vi "Textures Control.vi"(10 "Trial In Progress IN":T1, 11 "Trial Fraction IN":dbl) -> (2 "Left Texture Control":bool, 3 "Right Texture Control":bool)   [LabVIEW 2018]
uses:
  controls/Trial Config Settings.ctl
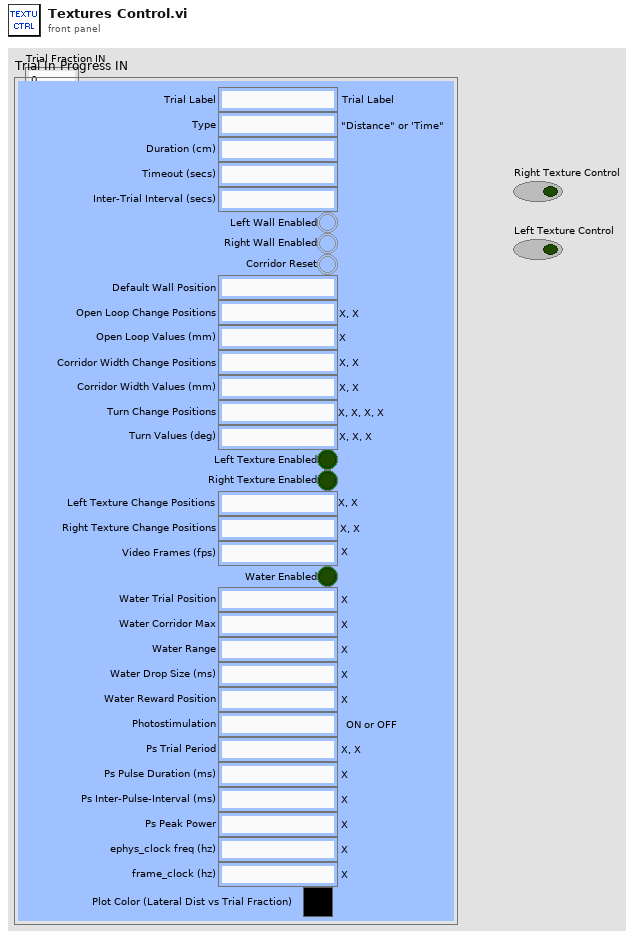
[diagram p1: front panel]
types:
  T1 = typedef "Trial Config Settings.ctl" = cluster{"Trial Label":string, "Type":string, "Timeout (secs)":string, "Inter-Trial Interval (secs)":string, "Left Wall Enabled":bool, "Right Wall Enabled":bool, "Corridor Reset":bool, "Default Wall Position":string, "Open Loop Change Positions":string, "Open Loop Values (mm)":string, "Corridor Width Change Positions":string, "Corridor Width Values (mm) ":string, "Turn Change Positions":string, "Turn Values (deg)":string, "Left Texture Change Positions":string, "Right Texture Change Positions":string, "Video Frames (fps)":string, "Water Enabled":bool, "Water Trial Position":string, "Photostimulation":string, "Water Corridor Max":string, "Water Range":string, "Water Drop Size (ms)":string, "Water Reward Position":string, "Duration (cm)":string, "Left Texture Enabled":bool, "Right Texture Enabled":bool, "Ps Trial Period":string, "Ps Inter-Pulse-Interval (ms)":string, "Ps Peak Power":string, "Ps Pulse Duration (ms)":string, "ephys_clock freq (hz)":string, "frame_clock (hz)":string, "Plot Color (Lateral Dist vs Trial Fraction)":u32}
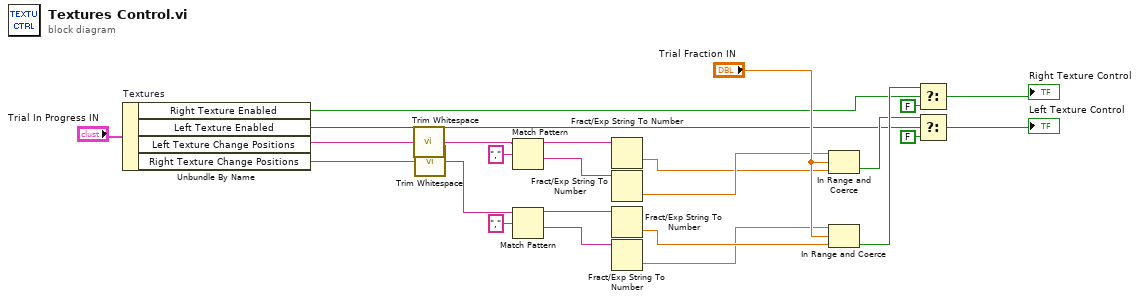
[diagram p0: block diagram]
diagram:
  n1 = Unbundle By Name "Textures"("Trial In Progress IN") -> ("Right Texture Enabled"=w1:bool, "Left Texture Enabled"=w2:bool, "Left Texture Change Positions"=w20:string, "Right Texture Change Positions"=w17:string)
  n2 = call <vilib>:"Trim Whitespace.vi"("string"=w20) -> ("trimmed string"=w19:string)  [unwired: 1 in]
  n3 = call <vilib>:"Trim Whitespace.vi"("string"=w17) -> ("trimmed string"=w18:string)  [unwired: 1 in]
  n4 = Match Pattern(string=w19, regular expression=",") -> (before substring=w6:string, after substring=w7:string)  [unwired: 1 in, 2 out]
  n5 = Match Pattern(string=w18, regular expression=",") -> (before substring=w14:string, after substring=w13:string)  [unwired: 1 in, 2 out]
  n6 = Fract/Exp String To Number(string=w6) -> (number=w8:dbl)  [unwired: 3 in, 1 out]
  n7 = Fract/Exp String To Number(string=w7) -> (number=w9:dbl)  [unwired: 3 in, 1 out]
  n8 = Fract/Exp String To Number(string=w14) -> (number=w12:dbl)  [unwired: 3 in, 1 out]
  n9 = Fract/Exp String To Number(string=w13) -> (number=w11:dbl)  [unwired: 3 in, 1 out]
  n10 = In Range and Coerce(upper limit=w9, x="Trial Fraction IN", lower limit=w8) -> (In Range?=w10:bool)  [unwired: 1 out]
  n11 = In Range and Coerce(upper limit=w11, x="Trial Fraction IN", lower limit=w12) -> (In Range?=w16:bool)  [unwired: 1 out]
  n12 = Select(t=w16, s=w1, f=FALSE ("Boolean")) -> (s? t:f=→"Right Texture Control":bool)
  n13 = Select(t=w10, s=w2, f=FALSE ("Boolean")) -> (s? t:f=→"Left Texture Control":bool)
